vi "receive.vi"(8 "error in (no error)":errorcluster, 9 "Batch Size In":i32, 10 "Queue Name in":string, 11 "RabbitMQ Session In":T1) -> (0 "error out":errorcluster, 1 "Message Array":string[](array[string]), 2 "Queue Name out":string, 3 "RabbitMQ Session Out":T1)   [LabVIEW 2019, in "rabbitmq.lvlib"]
uses:
  rabbitmq.lvlib
  session.ctl
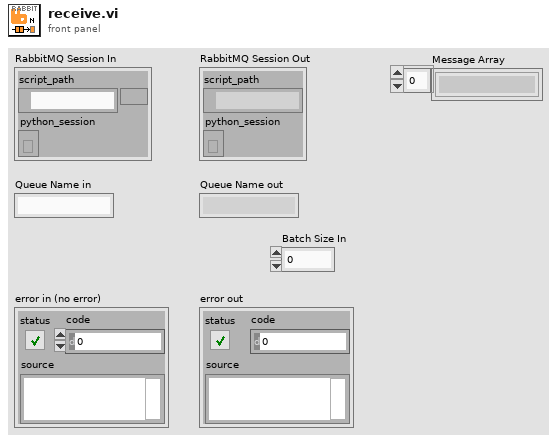
[diagram p1: front panel]
types:
  T1 = typedef "rabbitmq.lvlib/session.ctl" = cluster{"script_path":path, "python_session":refnum<k35>}
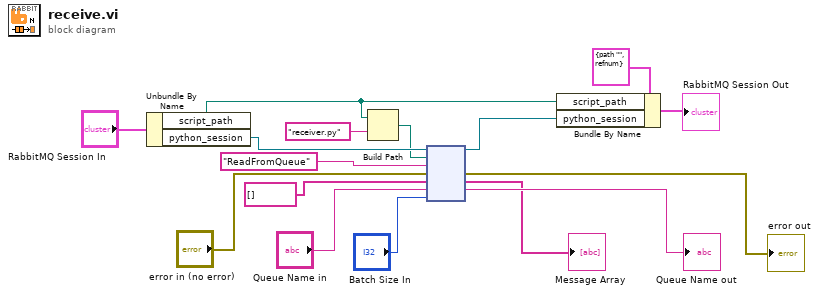
[diagram p0: block diagram]
diagram:
  n1 = Unbundle By Name("RabbitMQ Session In") -> ("script_path"=w5:path, "python_session"=w10:refnum<k35>)
  n2 = Build Path(base path=w5, name or relative path="receiver.py") -> (appended path=w4:path)
  n3 = node(w10, w4, "ReadFromQueue" ("function name"), "error in (no error)", string[] [], "Queue Name in", "Batch Size In") -> (w16:refnum<k35>, →"error out":errorcluster, →"Message Array":string[], →"Queue Name out":string)  [unwired: 1 in, 2 out]
  n4 = Bundle By Name(cluster=T1 {"script_path"=path "", "python_session"=refnum}, "script_path"=w5, "python_session"=w16) -> (→"RabbitMQ Session Out":T1)
